vi "Update Sensor Info.vi"(8 "error in (no error)":errorcluster, 10 "SensorInfo":refnum<class "SensorInfo.lvclass">, 11 "SensorView in":refnum<class "SensorView.lvclass">) -> (0 "error out":errorcluster, 3 "SensorView out":refnum<class "SensorView.lvclass">)   [LabVIEW 2012, in "Sensor Definition.lvlib" / "SensorView.lvclass"]
uses:
  SensorView.lvclass
  SensorInfo.lvclass
  SensorView.lvclass/SensorView.ctl
  Write SensorInfo.vi
  Read SensorInfo Changed Event.vi
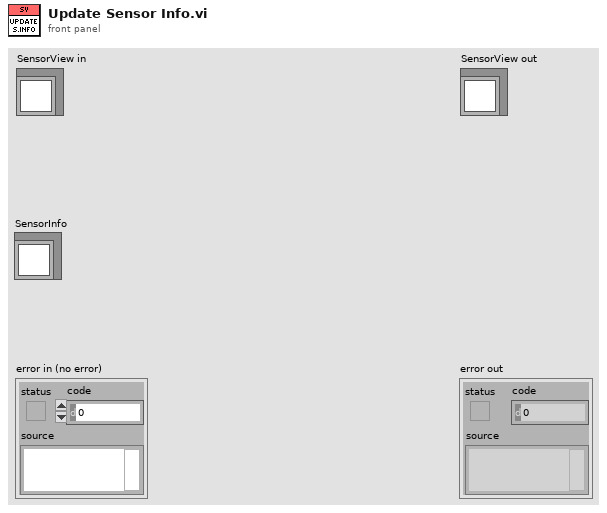
[diagram p1: front panel]
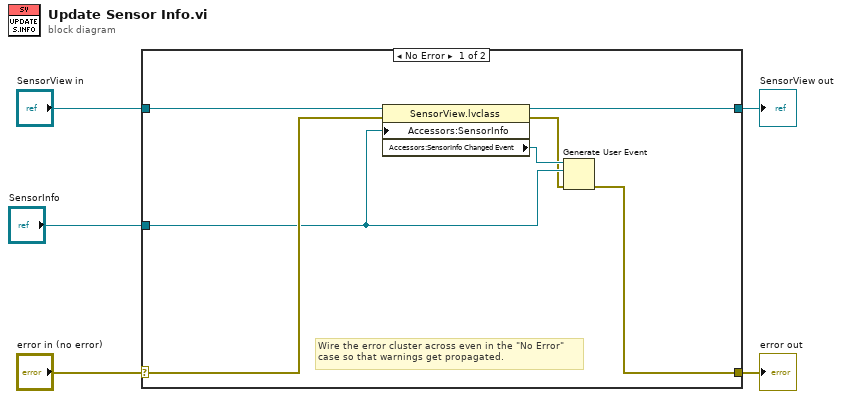
[diagram p0: block diagram]
diagram:
  n1 = case shown="No Error" "error in (no error)" {
    selector: "error in (no error)" -> [w10 w14]
    tunnel: [w6 w14] -> w4
    tunnel: [w11 w13] -> w2
    tunnel: "SensorView in" -> [w12 w13]
    tunnel: "SensorInfo" -> [w8 _]
    frame No Error {
      # "Wire the error cluster across even in the \"No Error\"\ncase so that warnings get propagated."
      n2 = property class="SensorView.lvclass"(reference=w12, error in=w10, "Accessors:SensorInfo"=w8) -> (reference out=w11:refnum<class "SensorView.lvclass">, error out=w7:errorcluster, "Accessors:SensorInfo Changed Event"=w9:refnum<user-event>)
      n3 = Generate User Event(user event=w9, event data cluster=w8, error in=w7) -> (error out=w6:errorcluster)  [unwired: 1 out]
    }
    frame Error {
    }
  }
  "error out" <- w4
  "SensorView out" <- w2
